vi "Test Error Propagation.vi"(11 "Test Case In":refnum<class "Test Open Xml.lvclass">) -> (0 "error out":errorcluster, 3 "Test Case Out":refnum<class "Test Open Xml.lvclass">)   [LabVIEW 2020, in "Test Open Xml.lvclass"]
uses:
  Test Open Xml.lvclass
  C:/Program Files/National Instruments/LabVIEW 2025/vi.lib/Astemes/LUnit/Test Case.lvclass
  <vilib>/Astemes/LUnit/Test Case.lvclass/Test Case.ctl
  5b340422-defb-4753-92ae-10f5ae7bb3d8.vi
  0ce37261-f17c-4487-8556-4dec27feb262.vi
  <vilib>/numeric/Random Number (Range) DBL.vi
  de3616c6-4837-4eef-92cf-f4a5127a2287.vi
  dbe47212-de57-4456-ba1d-2209d4b44483.vi
  4b527410-3829-466b-86c3-b8d1fd0707f5.vi
  a2e1416a-ebe4-4e53-9655-ad8087ccd270.vi
  f757fa54-b07b-4a92-a289-7ce739c836a6.vi
  de3616c6-4837-4eef-92cf-f4a5127a2287.vi/8154eede-cda4-41a2-91f5-d46003d40f50.vi
  <vilib>/Astemes/LUnit/Append Pass Result.vi
  <vilib>/Astemes/LUnit/Append Fail Result.vi
  f757fa54-b07b-4a92-a289-7ce739c836a6.vi/9c5d11cd-9439-4240-a1ee-d9baace9c924.vi
  <vilib>/Astemes/LUnit/Run In UI.vi
  <vilib>/Utility/error.llb/Clear Errors.vi
  Source/Get WorksheetPart.vi
  Source/Get or Add Cell.vi
  Source/Create CellValue.vi
  Source/Set CellValue.vi
  Source/Set Cell DataType.vi
  Source/Get or Add SharedStringTablePart.vi
  Source/Insert SharedString.vi
  Source/Timestamp to Excel Serial Date.vi
  Source/Set CellFormat to DateTime.vi
  Source/Open Xml.lvlib
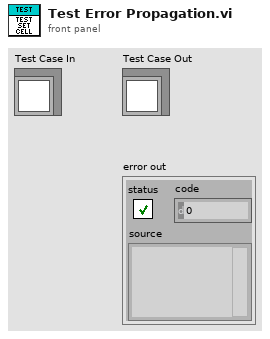
[diagram p1: front panel]
types:
  T1 = enum16{"Boolean", "Number", "Error", "SharedString", "String", "InlineString", "Date"}
  T2 = enum16{"Boolean", "Number", "Error", "SharedString", "String", "InlineString", "Date"}[]
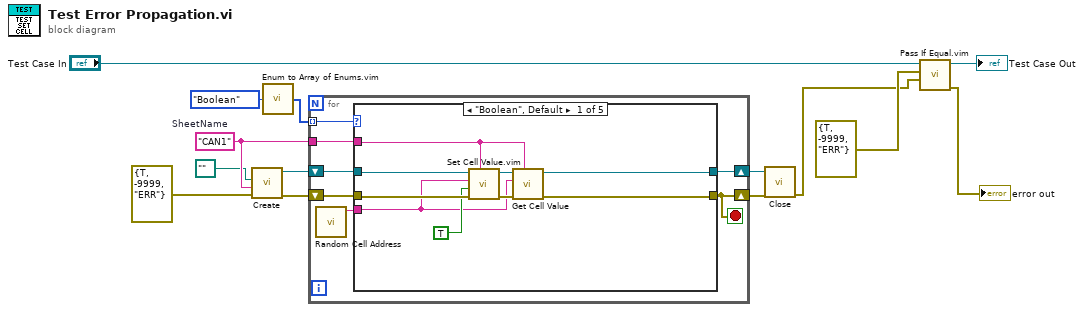
[diagram p0: block diagram]
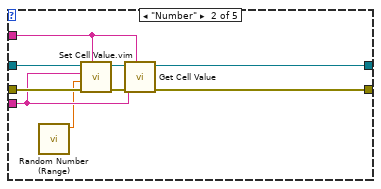
[diagram p2: hidden frame]
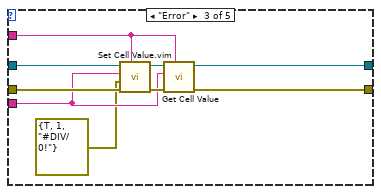
[diagram p3: hidden frame]
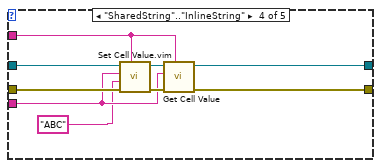
[diagram p4: hidden frame]
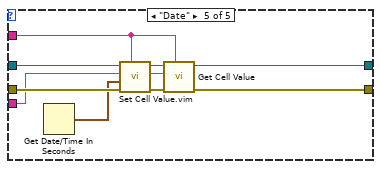
[diagram p5: hidden frame]
diagram:
  w7 = "CAN1"  # SheetName
  n1 = call "Create.vi"("error in"=errorcluster {"status"=TRUE, "code"=-9999, "source"="ERR"}, "SheetName"=w7, "Path"=path "") -> ("error out"=w10:errorcluster, "SpreadsheetDoc"=w11:refnum<k24>)  [unwired: 7 in]
  n2 = call "Enum to Array of Enums.vim"("enum"=T1."Boolean") -> ("array of enums"=w5:T2)
  n3 = for {
    tunnel: w7 -> [w18]
    shift-right: [w19] -> w8
    shift-left: w11 -> [w21]
    shift-right: [w16] -> w9
    shift-left: w10 -> [w20]
    tunnel: w5 -> [w17] mode=indexing
    stop <- w16 stop-if-true
    n4 = call "Random Cell Address.vi"() -> ("Random Cell Address"=w15:string)  [unwired: 11 in]
    n5 = case shown="\"Boolean\", Default" w17 {
      tunnel: w21 -> [w27 w39 w48 w57 w66]
      tunnel: w20 -> [w26 w38 w47 w56 w65]
      tunnel: [w24 w36 w45 w54 w63] -> w16
      tunnel: [w23 w34 w43 w52 w61] -> w19
      tunnel: w18 -> [w28 w33 w42 w51 w60]
      tunnel: w15 -> [w22 w32 w41 w50 w59]
      frame "Boolean", Default {
        n6 = call "Set Cell Value.vim"("Sheet Name"=w28, "error in"=w26, "Value"=TRUE, "Cell Address"=w22, "SpreadsheetDoc in"=w27) -> ("error out"=w30:errorcluster, "SpreadsheetDoc out"=w29:refnum<k24>)  [unwired: 5 in]
        n7 = call "Get Cell Value.vi"("Sheet Name"=w28, "error in"=w30, "Cell Address"=w22, "SpreadsheetDoc in"=w29) -> ("error out"=w24:errorcluster, "SpreadsheetDoc out"=w23:refnum<k24>)  [unwired: 4 in, 2 out]
      }
      frame "Number" {
        n8 = call-poly <vilib>:"Random Number (Range).vi"() -> ("number"=w31:dbl)  [unwired: 11 in]
        n9 = call "Set Cell Value.vim"("Sheet Name"=w33, "error in"=w38, "Value"=w31, "Cell Address"=w32, "SpreadsheetDoc in"=w39) -> ("error out"=w37:errorcluster, "SpreadsheetDoc out"=w35:refnum<k24>)  [unwired: 5 in]
        n10 = call "Get Cell Value.vi"("Sheet Name"=w33, "error in"=w37, "Cell Address"=w32, "SpreadsheetDoc in"=w35) -> ("error out"=w36:errorcluster, "SpreadsheetDoc out"=w34:refnum<k24>)  [unwired: 4 in, 2 out]
      }
      frame "Error" {
        n11 = call "Set Cell Value.vim"("Sheet Name"=w42, "error in"=w47, "Value"=errorcluster {"status"=TRUE, "code"=1, "source"="#DIV/0!"} ("error constant"), "Cell Address"=w41, "SpreadsheetDoc in"=w48) -> ("error out"=w46:errorcluster, "SpreadsheetDoc out"=w44:refnum<k24>)  [unwired: 5 in]
        n12 = call "Get Cell Value.vi"("Sheet Name"=w42, "error in"=w46, "Cell Address"=w41, "SpreadsheetDoc in"=w44) -> ("error out"=w45:errorcluster, "SpreadsheetDoc out"=w43:refnum<k24>)  [unwired: 4 in, 2 out]
      }
      frame "SharedString".."InlineString" {
        n13 = call "Set Cell Value.vim"("Sheet Name"=w51, "error in"=w56, "Value"="ABC", "Cell Address"=w50, "SpreadsheetDoc in"=w57) -> ("error out"=w55:errorcluster, "SpreadsheetDoc out"=w53:refnum<k24>)  [unwired: 5 in]
        n14 = call "Get Cell Value.vi"("Sheet Name"=w51, "error in"=w55, "Cell Address"=w50, "SpreadsheetDoc in"=w53) -> ("error out"=w54:errorcluster, "SpreadsheetDoc out"=w52:refnum<k24>)  [unwired: 4 in, 2 out]
      }
      frame "Date" {
        n15 = Get Date/Time In Seconds() -> (seconds since 1Jan1904=w58:timestamp)
        n16 = call "Set Cell Value.vim"("Sheet Name"=w60, "error in"=w65, "Value"=w58, "Cell Address"=w59, "SpreadsheetDoc in"=w66) -> ("error out"=w64:errorcluster, "SpreadsheetDoc out"=w62:refnum<k24>)  [unwired: 5 in]
        n17 = call "Get Cell Value.vi"("Sheet Name"=w60, "error in"=w64, "Cell Address"=w59, "SpreadsheetDoc in"=w62) -> ("error out"=w63:errorcluster, "SpreadsheetDoc out"=w61:refnum<k24>)  [unwired: 4 in, 2 out]
      }
    }
  }
  n18 = call "Close.vi"("error in"=w9, "SpreadsheetDoc"=w8) -> ("error out"=w3:errorcluster)  [unwired: 9 in]
  n19 = call "Pass If Equal.vim"("Actual"=w3, "Expected"=errorcluster {"status"=TRUE, "code"=-9999, "source"="ERR"} ("error constant"), "LUnit Test Case In"="Test Case In") -> ("error out"=→"error out":errorcluster, "LUnit Test Case Out"=→"Test Case Out":refnum<class "Test Open Xml.lvclass">)  [unwired: 7 in]
